vi "rotateXY.vi"(3 "B":dbl format="%#_13g", 4 "A":dbl format="%#_13g", 5 "theta":dbl format="%#_13g") -> (0 "Y":dbl, 1 "X":dbl)   [LabVIEW 2017]
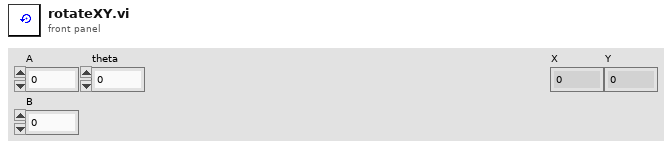
[diagram p1: front panel]
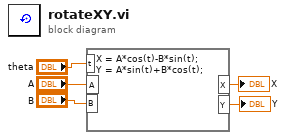
[diagram p0: block diagram]
diagram:
  n1 = formula code="X = A*cos(t)-B*sin(t);\nY = A*sin(t)+B*cos(t);"("t"="theta", "A"="A", "B"="B") -> ("X"=→"X":dbl, "Y"=→"Y":dbl)
